vi "SeCrTs-AI  Data  FGV.vi"(0 "Write/Read":T1=enum."Read", 5 "AI Channels Name LP":string[](array[string]), 7 "error in (no error)":errorcluster, 9 "AI Y LP data":dbl[](array[numeric]), 11 "AI LOX-LP data":waveform(dbl)[](array[waveform])) -> (6 "AI Channels Name LP":string[](array[string]), 8 "error Out":errorcluster, 10 "AI Y LP data":dbl[](array[numeric]), 15 "AI LOX-LP data":waveform(dbl)[](array[waveform]))   [LabVIEW 2022 SP3]
uses:
  RT Controls/SeCrTs-FGV Read write.ctl
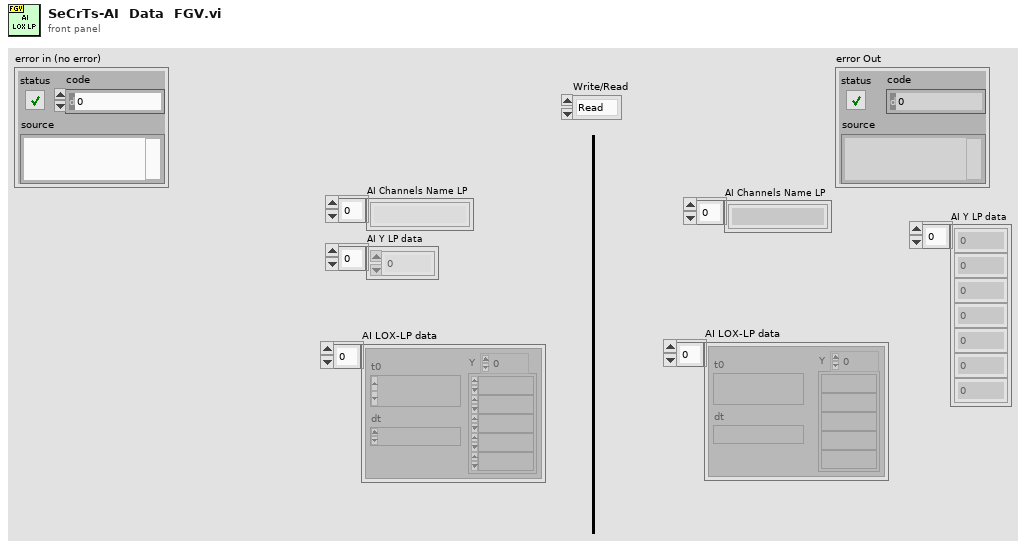
[diagram p1: front panel]
types:
  T1 = typedef "SeCrTs-FGV Read write.ctl" = enum16{"Write", "Read"}
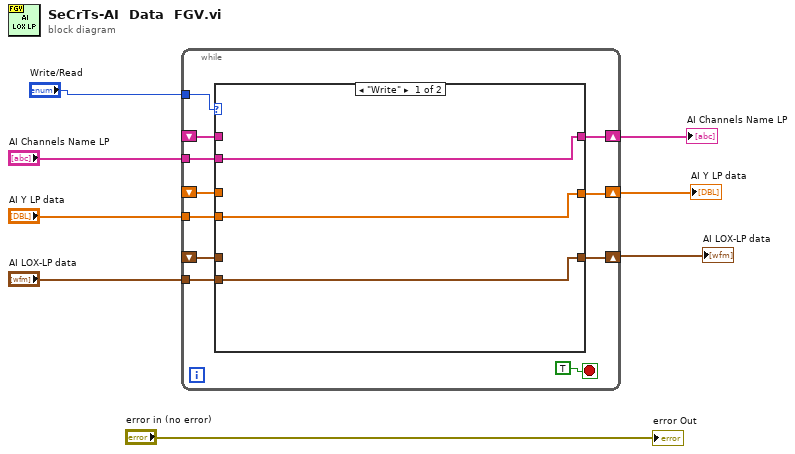
[diagram p0: block diagram]
diagram:
  n1 = while {
    tunnel: "Write/Read" -> [w18]
    shift-right: [w17] -> w7
    shift-left: _ -> [w16]
    shift-right: [w15] -> w5
    shift-left: _ -> [w14]
    shift-right: [w13] -> w3
    shift-left: _ -> [w12]
    tunnel: "AI Channels Name LP" -> [w11]
    tunnel: "AI Y LP data" -> [w10]
    tunnel: "AI LOX-LP data" -> [w9]
    stop <- TRUE stop-if-true
    n2 = case shown="\"Write\"" w18 {
      tunnel: [w22 w25] -> w17
      tunnel: w16 -> [_ w25]
      tunnel: [w21 w24] -> w15
      tunnel: w14 -> [_ w24]
      tunnel: [w20 w23] -> w13
      tunnel: w12 -> [_ w23]
      tunnel: w11 -> [w22 _]
      tunnel: w10 -> [w21 _]
      tunnel: w9 -> [w20 _]
      frame "Write" {
      }
      frame "Read" {
      }
    }
  }
  "AI Channels Name LP" <- w7
  "AI Y LP data" <- w5
  "AI LOX-LP data" <- w3
  "error Out" <- "error in (no error)"
